vi "DEMO.vi"() -> ()   [LabVIEW 2013]
uses:
  IP Adresss Control.xctl
panel:
  out "文本颜色":u32(colorbox)
  in  "获取文本颜色":bool
  out "Message":string
  in  "设置文本颜色":u32(colorbox)
  in  "IP Adresss Control":u32(xcontrol)
  out "IP":string
  in  "停止":bool
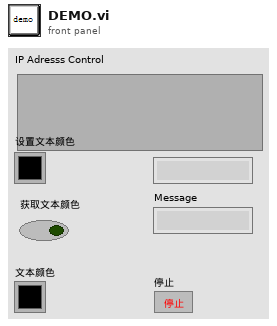
[diagram p1: front panel]
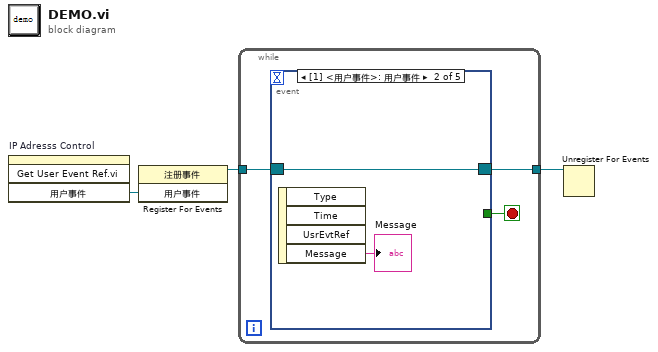
[diagram p0: block diagram]
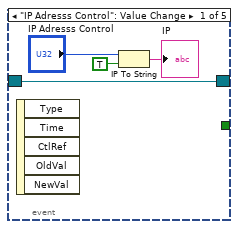
[diagram p2: hidden frame]
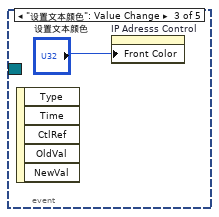
[diagram p3: hidden frame]
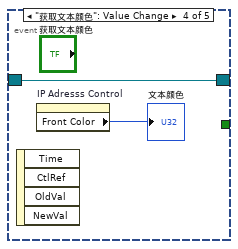
[diagram p4: hidden frame]
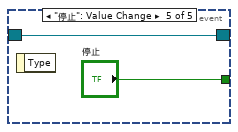
[diagram p5: hidden frame]
diagram:
  n1 = invoke on="IP Adresss Control" class="IP Adresss Control (严格)" method="Get User Event Ref.vi"() -> ("用户事件"=w1:refnum<user-event>)  [unwired: 4 in, 3 out]
  n2 = register-events(w1) -> (reference out=w3:refnum<event-registration>)  [unwired: 2 in, 1 out]
  n3 = while {
    tunnel: w3 -> [w5]
    tunnel: [w4] -> w2
    stop <- w6 stop-if-true
    n4 = event shown="[1] <用户事件>: 用户事件" {
      selector: w5 -> [w8 w12 _ w14 w16]
      dyn-events: [w8 w12 _ w14 w16] -> w4
      timeout: _ -> [_ _ _ _ _]
      tunnel: [_ _ _ _ "停止"] -> w6
      event "IP Adresss Control": Value Change {
        n5 = event-data() -> ()  [unwired: 1 in, 5 out]
        n6 = IP To String(1:TRUE ("句点符号？(F)"), 2:"IP Adresss Control") -> (0:→"IP":string)
      }
      event User Event {
        n7 = event-data() -> ("Message"=→"Message":string)  [unwired: 1 in, 3 out]
      }
      event "设置文本颜色": Value Change {
        n8 = event-data() -> ()  [unwired: 1 in, 5 out]
        n9 = property on="IP Adresss Control" class="IP Adresss Control (严格)"("Front Color"="设置文本颜色") -> ()  [unwired: 2 in, 2 out]
      }
      event "获取文本颜色": Value Change {
        n10 = event-data() -> ()  [unwired: 1 in, 4 out]
        n11 = property on="IP Adresss Control" class="IP Adresss Control (严格)"() -> ("Front Color"=→"文本颜色":u32)  [unwired: 2 in, 2 out]
      }
      event "停止": Value Change {
        n12 = event-data() -> ()  [unwired: 1 in, 1 out]
      }
    }
  }
  n13 = Unregister For Events(event registration refnum=w2) -> ()  [unwired: 1 in, 1 out]
